vi "SwerveJoystickLogic.vi"(0 "X":dbl, 5 "Y":dbl, 7 "Z":dbl, 9 "TankMode":bool, 11 "Gyro":dbl) -> (4 "Angles":dbl[](array[numeric]), 6 "Speeds":dbl[](array[numeric]))   [LabVIEW 2019]
uses:
  <vilib>/Rock Robotics/Network Tables/NT Read Boolean.vi
  Robot Global Data.vi
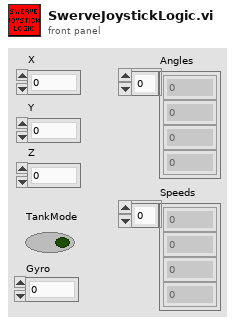
[diagram p1: front panel]
types:
  T1 = typedef "WPI_DriverStationRobotMode2.ctl" = enum16{"Autonomous Disabled", "Autonomous Enabled", "Teleop Disabled", "Teleop Enabled", "Disconnected", "Finish", "Test Disabled", "Test Enabled", "Emergency Stopped"}
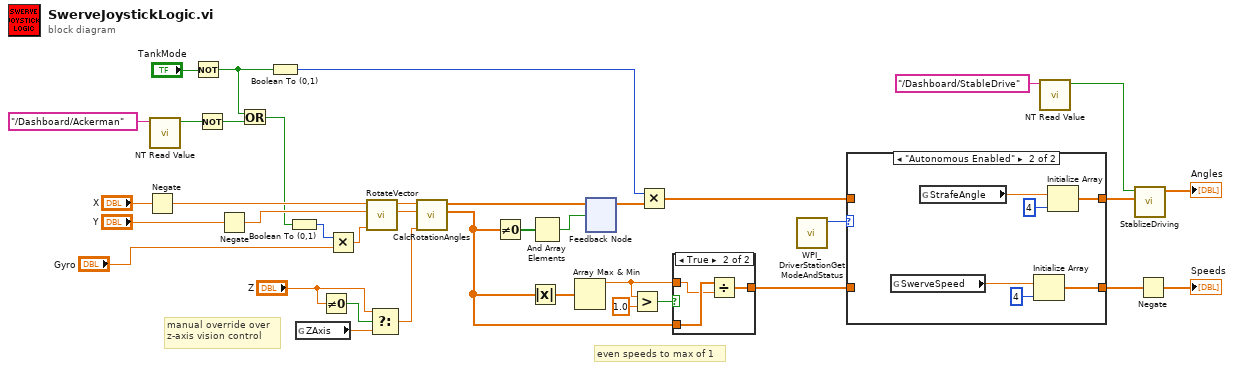
[diagram p0: block diagram]
diagram:
  # "even speeds to max of 1"
  # "manual override over\nz-axis vision control"
  n1 = Negate(x="X") -> (-x=w16:dbl)
  n2 = call-poly <vilib>:"NT Read Value.vi"("Name"="/Dashboard/Ackerman") -> ("Boolean"=w14:bool)  [unwired: 9 in, 1 out]
  n3 = Not(x="TankMode") -> (.not. x?=w13:bool)
  n4 = Not(x=w14) -> (.not. x?=w11:bool)
  n5 = Negate(x="Y") -> (-x=w20:dbl)
  n6 = Or(x=w13, y=w11) -> (x .or. y?=w12:bool)
  n7 = Boolean To (0,1)(Boolean=w13) -> (0, 1=w26:i16)
  n8 = Boolean To (0,1)(Boolean=w12) -> (0, 1=w15:i16)
  n9 = global read "Robot Global Data.vi" "ZAxis"() -> (w24:dbl)
  n10 = Not Equal To 0?(x="Z") -> (x != 0?=w25:bool)
  n11 = Multiply(x=w15, y="Gyro") -> (x*y=w28:dbl)
  n12 = call "RotateVector.vi"("Angle"=w28, "Y"=w20, "X"=w16) -> ("Y'"=w30:dbl, "X'"=w31:dbl)  [unwired: 6 in]
  n13 = Select(t="Z", s=w25, f=w24) -> (s? t:f=w6:dbl)
  n14 = call "CalcRotationAngles.vi"("ZAxis"=w6, "YAxis"=w30, "XAxis"=w31) -> ("Speeds"=w35:dbl[], "Angles"=w34:dbl[])  [unwired: 7 in]
  n15 = Not Equal To 0?(x=w35) -> (x != 0?=w32:bool[])
  n16 = Absolute Value(x=w35) -> (abs(x)=w36:dbl[])
  n17 = And Array Elements(Boolean array=w32) -> (logical AND=w33:bool)
  n18 = Array Max & Min(array=w36) -> (max value=w37:dbl)  [unwired: 3 out]
  n19 = feedback #1() -> (w27:dbl[])  [unwired: 1 in]
  n20 = feedback-in #1(w34, w33) -> ()
  n21 = Greater?(x=w37, y=1.0) -> (0:w18:bool)
  n22 = Multiply(x=w26, y=w27) -> (x*y=w23:dbl[])
  n23 = case shown="True" w18 {
    tunnel: w35 -> [w39 w42]
    tunnel: w37 -> [_ w41]
    tunnel: [w39 w40] -> w22
    frame False {
    }
    frame True {
      n24 = Divide(x=w42, y=w41) -> (x/y=w40:dbl[])
    }
  }
  n25 = call <vilib>:"WPI_DriverStationGetModeAndStatus.vi"() -> ("Robot Mode"=w21:T1)  [unwired: 10 in, 1 out]
  n26 = case shown="\"Autonomous Enabled\"" w21 {
    tunnel: w23 -> [w44 _]
    tunnel: [w44 w46] -> w3
    tunnel: [w43 w48] -> w4
    tunnel: w22 -> [w43 _]
    frame "Autonomous Disabled", Default {
    }
    frame "Autonomous Enabled" {
      n27 = global read "Robot Global Data.vi" "SwerveSpeed"() -> (w47:dbl)
      n28 = global read "Robot Global Data.vi" "StrafeAngle"() -> (w45:dbl)
      n29 = Initialize Array(w47, 4 ("dimension size")) -> (w48:dbl[])
      n30 = Initialize Array(w45, 4 ("dimension size")) -> (w46:dbl[])
    }
  }
  n31 = call-poly <vilib>:"NT Read Value.vi"("Name"="/Dashboard/StableDrive") -> ("Boolean"=w2:bool)  [unwired: 9 in, 1 out]
  n32 = call "StablizeDriving.vi"("AngleSetpoints"=w3, "Enable"=w2) -> ("NewAngles"=→"Angles":dbl[])  [unwired: 9 in]
  n33 = Negate(x=w4) -> (-x=→"Speeds":dbl[])
